vi "Parse_Definition.vi"(8 "error in (no error)":errorcluster, 11 "JSON String In":string) -> (0 "error out":errorcluster, 1 "Found?":bool, 2 "Definition(s)":string, 3 "JSON String Out":string)   [LabVIEW 2018, in "MerriamWebsterJSON.lvlib"]
uses:
  MerriamWebsterJSON.lvlib
  <vilib>/LVH/i3 JSON/JSON Parsing/Get Array Value at Index Files/Get Array Value at Index - Object.vi
  <vilib>/LVH/i3 JSON/JSON Parsing/Get Object Parameter Files/Get Object Parameter - Object.vi
  <vilib>/LVH/i3 JSON/JSON Parsing/Get Array Value at Index Files/Get Array Value at Index - String.vi
  <vilib>/LVH/i3 JSON/i3-json.lvlib
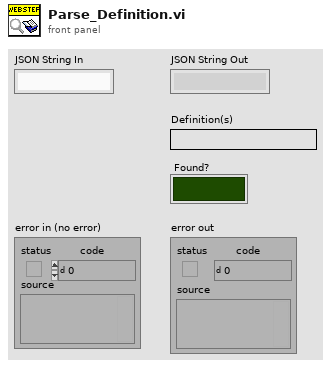
[diagram p1: front panel]
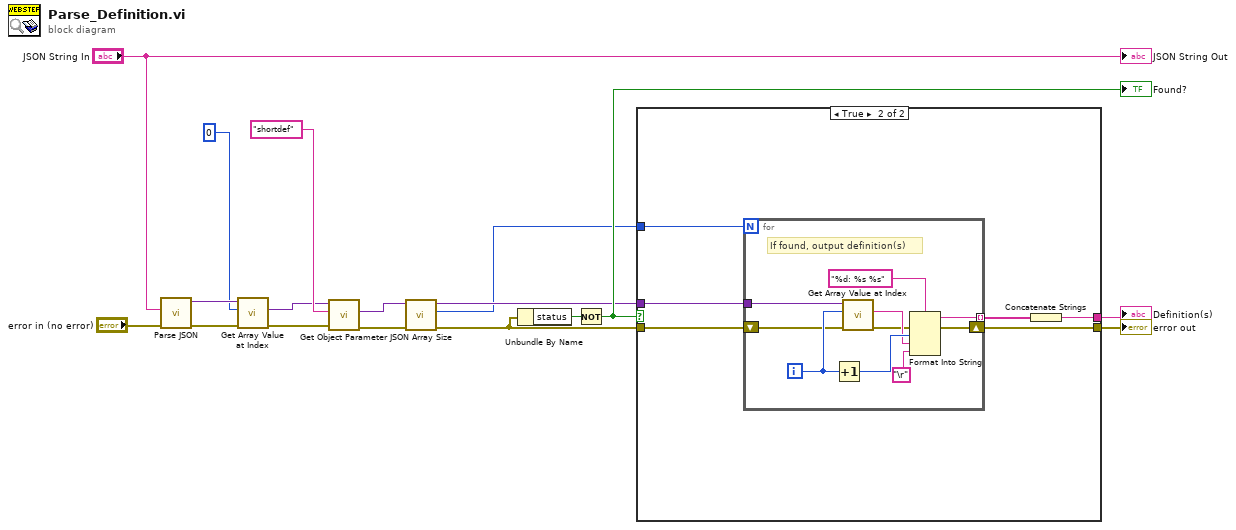
[diagram p0: block diagram]
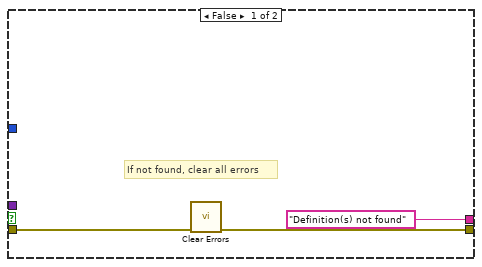
[diagram p2: hidden frame]
diagram:
  n1 = call <vilib>:"Parse JSON.vi"("error in (no error)"="error in (no error)", "JSON String"="JSON String In") -> ("error out"=w12:errorcluster, "JSON Tree"=w17:variant)  [unwired: 6 in, 2 out]
  n2 = call-poly <vilib>:"Get Array Value at Index.vi"("error in (no error)"=w12, "Index"=0, "JSON Tree In (JSON Array)"=w17) -> ("error out"=w9:errorcluster, "JSON Object"=w10:variant)  [unwired: 5 in, 2 out]
  n3 = call-poly <vilib>:"Get Object Parameter.vi"("error in (no error)"=w9, "Parameter Name"="shortdef", "JSON Tree In (JSON Object)"=w10) -> ("error out"=w14:errorcluster, "JSON Object"=w11:variant)  [unwired: 5 in, 2 out]
  n4 = call <vilib>:"JSON Array Size.vi"("error in (no error)"=w14, "JSON Tree In (JSON Array)"=w11) -> ("error out"=w3:errorcluster, "Array Size"=w1:i32, "JSON Tree Passthrough (JSON Array)"=w2:variant)  [unwired: 7 in]
  n5 = Unbundle By Name(w3) -> ("status"=w8:bool)
  n6 = Not(x=w8) -> (.not. x?=w7:bool)
  "Found?" <- w7
  n7 = case shown="True" w7 {
    tunnel: [w20 w23] -> w5
    tunnel: ["Definition(s) not found" ("String Value") w21] -> w6
    tunnel: w3 -> [w18 w24]
    tunnel: w2 -> [_ w26]
    tunnel: w1 -> [_ w25]
    frame False {
      # "If not found, clear all errors"
      n8 = call <vilib>:"Clear Errors.vi"("error in (no error)"=w18) -> ("error out"=w20:errorcluster)  [unwired: 5 in, 1 out]
    }
    frame True {
      n9 = for {
        N: w25 -> [_]
        tunnel: [w31] -> w22 mode=indexing
        tunnel: w26 -> [w29]
        shift-right: [w27] -> w23
        shift-left: w24 -> [w30]
        i -> [w35]
        # "If found, output definition(s)"
        n10 = Increment(x=w35) -> (x+1=w34:i32)
        n11 = call-poly <vilib>:"Get Array Value at Index.vi"("error in (no error)"=w30, "Index"=w35, "JSON Tree In (JSON Array)"=w29) -> ("error out"=w28:errorcluster, "String Value"=w33:string)  [unwired: 5 in, 2 out]
        n12 = Format Into String(format string="%d: %s %s", error in=w28, w34, w33, "\r") -> (resulting string=w31:string, error out=w27:errorcluster)  [unwired: 1 in]
      }
      n13 = Concatenate Strings(w22) -> (w21:string)
    }
  }
  "error out" <- w5
  "Definition(s)" <- w6
  "JSON String Out" <- "JSON String In"
